vi "Puma Ground Control Station Read Version.vi"() -> ()   [LabVIEW 2014]
doc: "The Advanced Serial Read and Write example performs a Serial Port Read, a Serial Port Write, or a combination of these actions while setting some advanced serial features like buffer size, termination characters, and XON/XOFF flow control. The user selects the actions (read or write) on the front panel. If both are selected, the VI will write the data first, read the data and then close the VISA session that is opened to the port. \n\nThe parameters set for the serial port must match the parameters of the connected instrument or device. In this example, the bytes to read parameter specifies the number of bytes that the serial port reads. If there were more bytes at the port than the number specified in bytes to read, those bytes would not be read. Also, if you specify to read more bytes than the number of bytes actually read, you might receive a timeout error message.\n\nINSTRUCTIONS:\n1) Select the serial resource and configuration parameters (baud rate, data bits, parity, stop bits, flow control).\n2) Termination character can be enabled and set. Also, set the required input buffer size prior to running the example.\n3) Select the operations to be performed. \n4) Connect the serial port to your device. If no device is available, perform a loopback test by doing one of the following. Short pins 2 and 3 on a RS-232 cable or short pin 4 to pin 8 and pin 5 to pin 9 on a RS-485/422 cable. \n5) Run the VI to see the data read. (The \"read string\" will match the \"string to write\" if a loopback test was performed.)\n\nThis example exposes several advanced features that you may need for your application. Not all applications need all the features shown in this example. The input buffer size is likely an important setting that you want to control in your application. This example expands upon the flow control option for XON and XOFF, allowing the user to choose those control characters. The timeout parameter has been brought to the front panel so a user can specify the time period the VISA Read will wait for the number of bytes to read before timing out. Also, the user has several controls for the termination character, which is discussed later.\n\nNote that you can press the write and read buttons and change the bytes to read parameters on the fly, while the example is running. However, you must stop the example to change the other configuration parameters after the example has started running, and then run again.\n\nSet the I/O buffer size slightly higher the amount of data you expect to receive. This is very important for applications that don't use flow control, as you may lose characters if the receive buffer overflows.\n\nSetting the timeout period ensures that the operation returns with a timeout error if the operation cannot be performed in the specified time period. \n\nSome devices require a termination character in order to identify the end of command strings. Some devices send a termination character to signify the end of data to be read. \n\nThis example shows how you can end the Read operation once a termination character is detected in the buffer and/or append a termination character at the end of the Write data. To enable the Read to end on a termination character, use the VISA Configure Serial Port or use the VISA Properties Serial End Mode for Reads, Termination Character Enable, and Termination Character. To end the Write with a termination character, use the VISA Properties Serial End Mode for Writes, the Send End Enable, and Termination Character. In this example, the same termination character is used for both the Read and the Write. You can specify two different characters for your application, if desired.\n\nYour application may require specific characters for the XON/XOFF Flow Control. You can specify these characters with the VISA Properties Flow Control XOFF Character and Flow Control XON Character. Note that if the standard XON and XOFF characters are used, then decimal 17 and 19 are unavailable for data values. Remember that using flow control and setting an adequate buffer size allow you to prevent buffer overflows."
panel:
  out "soft kill ind":bool
  out "dump fuel ind":bool
  out "abort ind":bool
  out "run ind":bool
  out "av6-t ind":bool
  out "Control input":bool
  out "return yes on a completed input":bool
  out "Control (on/off)":bool
  out "PT 7":dbl
  out "PT7":dbl
  out "PT6":dbl
  out "PT5":dbl
  out "PT4":dbl
  out "PT3":dbl
  out "PT2":dbl
  out "PT1":dbl
  out "TC6":dbl
  out "TC5":dbl
  out "TC4":dbl
  out "TC3":dbl
  out "TC2":dbl
  out "TC1":dbl
  out "Output":string
  in  "?":enum32{"Check Out's", "Test"}(tab)
  in  "Tank ISO / AV5-T":bool
  in  "DValve / AV6-T":bool
  in  "Ullage ISO / FC-U":bool
  in  "Safety":bool
  in  "Test Run":bool
  in  "Reset Control":bool
  out "?":bool
  out "?":bool
  out "?":bool
  out "?":bool
  in  "Soft Kill":bool
  in  "Reset FC":bool
  in  "Safety":bool
  in  "Takeoff":bool
  in  "abort":bool
  out "?":dbl(graph)
  out "?":string[](array[string])
  out "?":string[](array[string])
  out "?":T1(graph)
  out "Voltage Sensor":dbl
  out "PT 1":dbl
  out "PT 2":dbl
  out "PT 3":dbl
  out "PT 4":dbl
  out "PT 5":dbl
  out "PT 6":dbl
  out "TC 1":dbl
  out "TC 2":dbl
  out "TC 3":dbl
  out "TC 4":dbl
  out "TC 5":dbl
  out "TC 6":dbl
  in  "dump fuel":bool
  in  "?":enum32{"PT", "TC", "Test"}(tab)
  in  "?":T2(tab)
  out "PT 1":dbl(graph)
  out "PT 2":dbl(graph)
  out "PT 3":dbl(graph)
  out "PT 4":dbl(graph)
  out "PT 5":dbl(graph)
  out "PT 6":dbl(graph)
  out "PT 7":dbl(graph)
  in  "?":T3(tab)
  out "TC 1":dbl(graph)
  out "TC 2":dbl(graph)
  out "TC 3":dbl(graph)
  out "TC 4":dbl(graph)
  out "TC 5":dbl(graph)
  out "TC 6":dbl(graph)
  out "?":bool
  out "String":string
  in  "String 3":string
  in  "Turn Off":bool
  in  "?":bool
  in  "Av-6Tt":bool
  in  "?":bool
  out "AV4-T":bool
  out "AV3-T":bool
  out "AV2-T":bool
  out "AV1-T":bool
  out "AV6-T":bool
  out "AV5-T":bool
  out "FO-U":bool
  out "FC-U":bool
  out "?":dbl(slide) scale=0.2..200.0
  # "FC-U"
  # "FO-U"
  # "AV1-T"
  # "AV2-T"
  # "AV3-T"
  # "AV4-T"
  # "AV5-T"
  # "AV6-T"
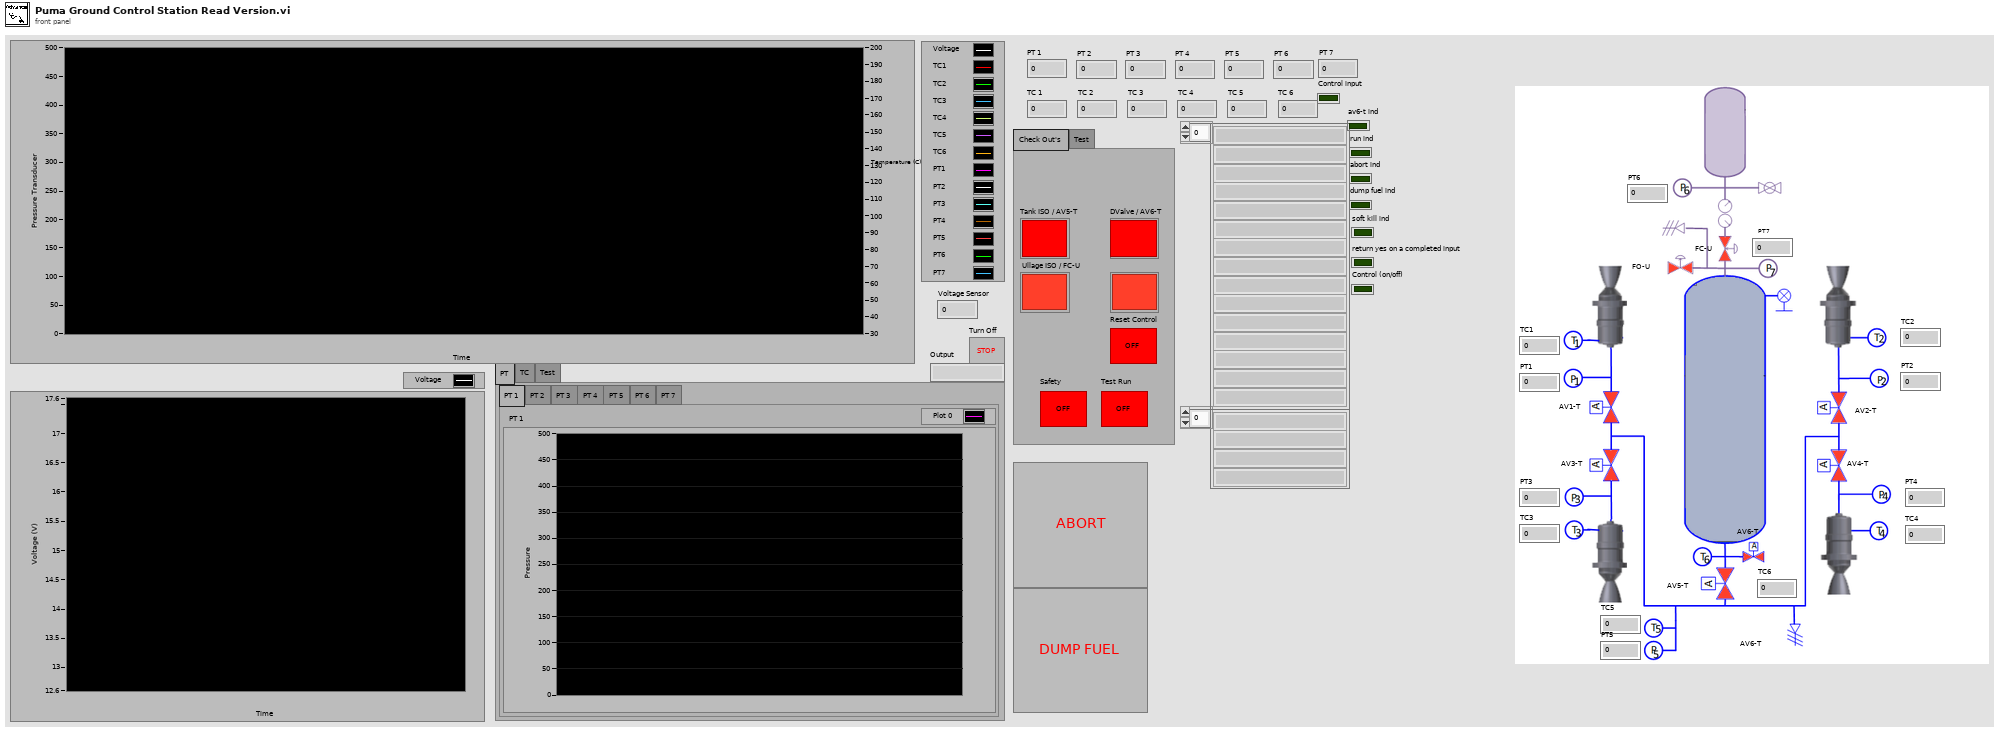
[diagram p1: front panel]
types:
  T1 = cluster{dbl, dbl, dbl, dbl, dbl, dbl, dbl, dbl, dbl, dbl, dbl, dbl, dbl, dbl}
  T2 = enum32{"PT 1", "PT 2", "PT 3", "PT 4", "PT 5", "PT 6", "PT 7"}
  T3 = enum32{"TC 1", "TC 2", "TC 3", "TC 4", "TC 5", "TC 6"}
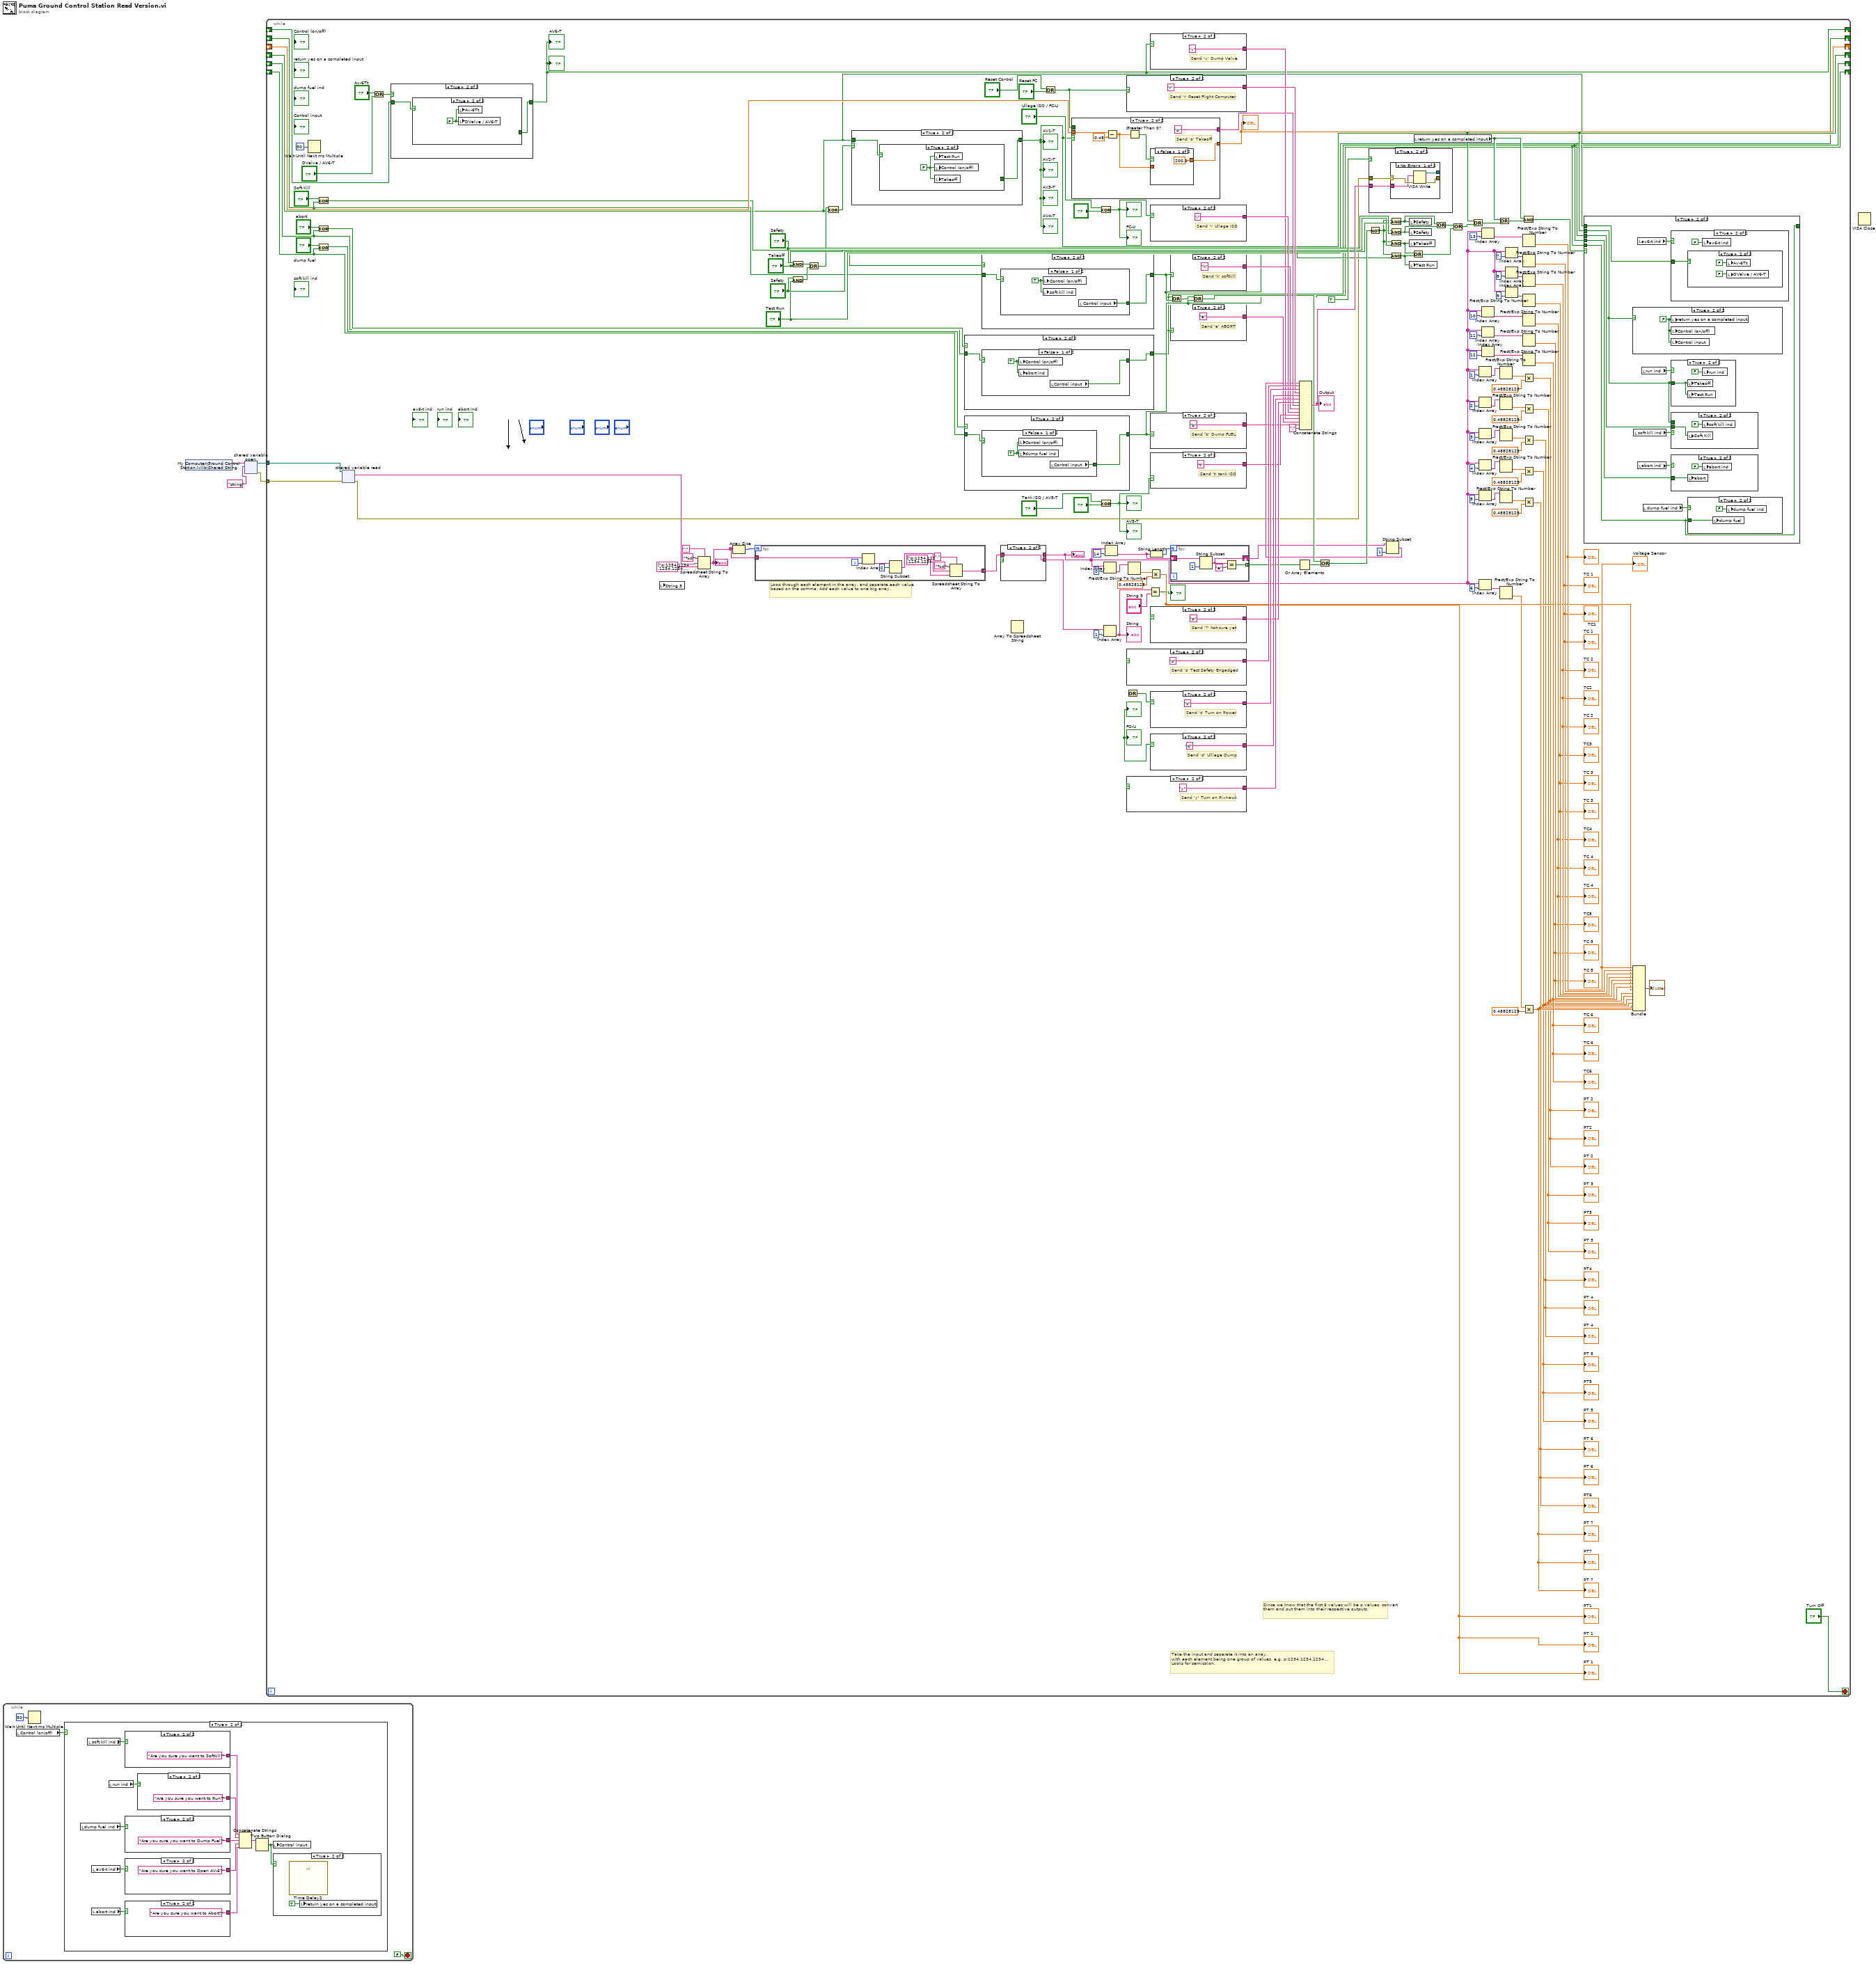
[diagram p0: block diagram]
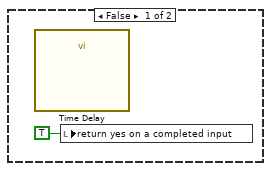
[diagram p8: hidden frame]
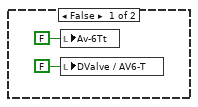
[diagram p11: hidden frame]
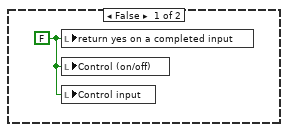
[diagram p16: hidden frame]
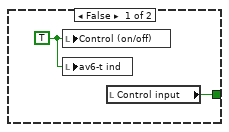
[diagram p18: hidden frame]
diagram:
  n1 = while {
    stop <- FALSE stop-if-true
    n2 = local read "Control (on/off)"() -> (w7:bool)
    n3 = Wait Until Next ms Multiple(millisecond multiple=u32 50 ("milliseconds to wait")) -> ()  [unwired: 1 out]
    n4 = case shown="True" w7 {
      frame False {
      }
      frame True {
        n5 = local read "dump fuel ind"() -> (w16:bool)
        n6 = local read "soft kill ind"() -> (w14:bool)
        n7 = local read "av6-t ind"() -> (w17:bool)
        n8 = local read "abort ind"() -> (w18:bool)
        n9 = local read "run ind"() -> (w15:bool)
        n10 = case shown="True" w14 {
          tunnel: [_ "Are you sure you want to Softkill?"] -> w9
          frame False {
          }
          frame True {
          }
        }
        n11 = case shown="True" w16 {
          tunnel: [_ "Are you sure you want to Dump Fuel?"] -> w11
          frame False {
          }
          frame True {
          }
        }
        n12 = case shown="True" w17 {
          tunnel: [_ "Are you sure you want to Open AV-6?"] -> w12
          frame False {
          }
          frame True {
          }
        }
        n13 = case shown="True" w18 {
          tunnel: [_ "Are you sure you want to Abort?"] -> w13
          frame False {
          }
          frame True {
          }
        }
        n14 = case shown="True" w15 {
          tunnel: [_ "Are you sure you want to Run?"] -> w10
          frame False {
          }
          frame True {
          }
        }
        n15 = Concatenate Strings(w9, w10, w11, w12, w13) -> (w8:string)
        n16 = Two Button Dialog(message=w8) -> (T button?=w19:bool)  [unwired: 2 in]
        n17 = local write "Control input"(w19) -> ()
        n18 = case shown="True" w19 {
          frame False {
            n19 = call "Time Delay"() -> ()  [unwired: 11 in, 1 out]
            n20 = local write "return yes on a completed input"(TRUE) -> ()
          }
          frame True {
            n21 = call "Time Delay2"() -> ()  [unwired: 11 in, 1 out]
            n22 = local write "return yes on a completed input"(TRUE) -> ()
          }
        }
      }
    }
  }
  n23 = shared-variable "My Computer\\Ground Control Station.lvlib\\Shared String"() -> (w4:string)  [unwired: 1 in, 1 out]
  n24 = shared-variable-open(w4, "string") -> (w2:refnum<k21>, w1:errorcluster)  [unwired: 2 in]
  n25 = while {
    shift-right: [w115] -> _
    shift-left: _ -> [w114]
    shift-right: [w56] -> _
    shift-left: _ -> [w38]
    shift-right: [w46] -> _
    shift-left: _ -> [w47]
    shift-right: [w36] -> _
    shift-left: _ -> [w63]
    shift-right: [w37] -> _
    shift-left: _ -> [w60]
    shift-right: [w39] -> _
    shift-left: _ -> [w42]
    tunnel: w2 -> [w30]
    tunnel: w1 -> [w27]
    stop <- "Turn Off" stop-if-true
    # "Since we know that the first 6 values will be p values, convert them and put them into their respective outputs."
    # "Loop through each element in the array, and separate each value\nbased on the comma. Add each value to one big array."
    # "Take the input and separate it into an array,\nwith each element being one group of values, e.g. p:1234,1234,1234...\nLooks for semicolon."
    n26 = Wait Until Next ms Multiple(millisecond multiple=u32 50 ("milliseconds to wait")) -> ()  [unwired: 1 out]
    n27 = Exclusive Or(1:w42, 2:"Soft Kill") -> (0:w40:bool)
    n28 = Exclusive Or(1:w63, 2:"abort") -> (0:w65:bool)
    n29 = Exclusive Or(1:w60, 2:"dump fuel") -> (0:w62:bool)
    n30 = shared-variable-read(w30, w27) -> (w28:errorcluster, w29:string)  [unwired: 2 out]
    n31 = Or(x="Av-6Tt", y="DValve / AV6-T") -> (x .or. y?=w43:bool)
    n32 = case shown="True" w43 {
      tunnel: [w207 w208] -> w46
      tunnel: w47 -> [w207 w209]
      frame False {
      }
      frame True {
        n33 = case shown="True" w209 {
          tunnel: [w211 _] -> w208
          frame False {
            w210 = TRUE
            n34 = local write "Control (on/off)"(w210) -> ()
            n35 = local write "av6-t ind"(w210) -> ()
            n36 = local read "Control input"() -> (w211:bool)
          }
          frame True {
            w212 = FALSE
            n37 = local write "Av-6Tt"(w212) -> ()
            n38 = local write "DValve / AV6-T"(w212) -> ()
          }
        }
      }
    }
    "AV6-T" <- w46
    "?" <- w46
    n39 = local read "String 3"() -> ()  [unwired: 1 in]
    n40 = Spreadsheet String To Array(delimiter (Tab)=";", format string="%d", spreadsheet string=w29, array type (2D Dbl)=string[] ["p:1234.1234.1234.1234,1234,1234", "t:1234,1234,1234"] ("Array of Strings 3")) -> (array=w173:string[])
    "?" <- w173
    n41 = Array Size(array=w173) -> (size(s)=w174:i32)
    n42 = for {
      N: w174 -> [_]
      tunnel: w173 -> [w282]
      tunnel: [w274] -> w84 mode=concatenating
      i -> [w281]
      n43 = Index Array(array=w282, index=w281) -> (element=w277:string)
      n44 = String Subset(string=w277, offset (0)=2) -> (substring=w275:string)  [unwired: 1 in]
      n45 = Spreadsheet String To Array(delimiter (Tab)=",", format string="%d", spreadsheet string=w275, array type (2D Dbl)=string[] ["p:1234.1234.1234.1234,1234,1234", "t:1234,1234,1234"] ("Array of Strings 3")) -> (array=w274:string[])
    }
    n46 = And(x="Safety", y="Takeoff") -> (x .and. y?=w133:bool)
    n47 = And(x="Safety", y="Test Run") -> (x .and. y?=w134:bool)
    n48 = Or(x=w133, y=w134) -> (x .or. y?=w68:bool)
    n49 = Exclusive Or(1:w38, 2:w68) -> (0:w67:bool)
    n50 = case shown="True" w67 {
      tunnel: [w229 w231] -> w56
      tunnel: w38 -> [w229 w230]
      frame False {
      }
      frame True {
        n51 = case shown="True" w230 {
          tunnel: [w233 _] -> w231
          frame False {
            w232 = TRUE
            n52 = local write "Control (on/off)"(w232) -> ()
            n53 = local write "run ind"(w232) -> ()
            n54 = local read "Control input"() -> (w233:bool)
          }
          frame True {
            w234 = FALSE
            n55 = local write "Test Run"(w234) -> ()
            n56 = local write "Control (on/off)"(w234) -> ()
            n57 = local write "Takeoff"(w234) -> ()
          }
        }
      }
    }
    "AV1-T" <- w56
    "AV4-T" <- w56
    "AV2-T" <- w56
    "AV3-T" <- w56
    n58 = case shown="True" w65 {
      tunnel: [w223 w225] -> w36
      tunnel: w63 -> [w223 w224]
      frame False {
      }
      frame True {
        n59 = case shown="False" w224 {
          tunnel: [w226 FALSE ("T button?")] -> w225
          frame False {
            w227 = TRUE
            n60 = local write "Control (on/off)"(w227) -> ()
            n61 = local write "abort ind"(w227) -> ()
            n62 = local read "Control input"() -> (w226:bool)
          }
          frame True {
          }
        }
      }
    }
    n63 = case shown="True" w62 {
      tunnel: [w218 w220] -> w37
      tunnel: w60 -> [w218 w219]
      frame False {
      }
      frame True {
        n64 = case shown="False" w219 {
          tunnel: [w222 _] -> w220
          frame False {
            w221 = TRUE
            n65 = local write "Control (on/off)"(w221) -> ()
            n66 = local write "dump fuel ind"(w221) -> ()
            n67 = local read "Control input"() -> (w222:bool)
          }
          frame True {
          }
        }
      }
    }
    n68 = case shown="True" w40 {
      tunnel: [w213 w215] -> w39
      tunnel: w42 -> [w213 w214]
      frame False {
      }
      frame True {
        n69 = case shown="False" w214 {
          tunnel: [w216 _] -> w215
          frame False {
            w217 = TRUE
            n70 = local write "Control (on/off)"(w217) -> ()
            n71 = local write "soft kill ind"(w217) -> ()
            n72 = local read "Control input"() -> (w216:bool)
          }
          frame True {
          }
        }
      }
    }
    n73 = case shown="True" {
      selector: _ -> [_ _]
      tunnel: w84 -> [w240 w241]
      tunnel: [w240 _] -> w85
      tunnel: [_ w241] -> w83
      frame False {
      }
      frame True {
      }
    }
    "?" <- w85
    n74 = Array To Spreadsheet String() -> ()  [unwired: 3 in, 1 out]
    n75 = Or(x="Reset Control", y="Reset FC") -> (x .or. y?=w116:bool)
    n76 = case shown="True" w56 {
      tunnel: [_ "o" ("write buffer")] -> w138
      tunnel: w114 -> [w251 w259]
      tunnel: [w252 w255] -> w115
      tunnel: w116 -> [w250 _]
      frame False {
        n77 = case shown="False" w250 {
          tunnel: [w253 200.0] -> w252
          tunnel: w251 -> [w253 _]
          frame False {
          }
          frame True {
          }
        }
      }
      frame True {
        # "Send 'o' Takeoff"
        n78 = Subtract(x=w259, y=0.48) -> (x-y=w256:dbl)
        n79 = Greater Than 0?(x=w256) -> (x > 0?=w257:bool)
        n80 = case shown="False" w257 {
          tunnel: w256 -> [_ w262]
          tunnel: [200.0 w262] -> w255
          frame False {
          }
          frame True {
          }
        }
      }
    }
    "?" <- w115
    n81 = Exclusive Or(1:"?", 2:"Ullage ISO / FC-U") -> (0:w107:bool)
    "FC-U" <- w107
    "?" <- w107
    n82 = Exclusive Or(1:"?", 2:"Tank ISO / AV5-T") -> (0:w110:bool)
    "AV5-T" <- w110
    "?" <- w110
    n83 = Index Array(array=w85, index=0) -> (element=w166:string)
    n84 = Index Array(array=w83, index=1) -> (element=w82:string)
    "String" <- w82
    n85 = Index Array(array=w85, index=14) -> (element=w31:string)
    n86 = case shown="True" w116 {
      tunnel: [_ "r" ("write buffer")] -> w142
      frame False {
      }
      frame True {
        # "Send 'r' Reset Flight Computer"
      }
    }
    n87 = case shown="True" {
      selector: _ -> [_ _]
      tunnel: [_ "s" ("write buffer")] -> w145
      frame False {
      }
      frame True {
        # "Send 's' Test Safety Engadged"
      }
    }
    n88 = case shown="True" {
      selector: _ -> [_ _]
      tunnel: [_ "y" ("write buffer")] -> w140
      frame False {
      }
      frame True {
        # "Send 'y' Turn on Pixhawk"
      }
    }
    n89 = Or() -> (x .or. y?=w132:bool)  [unwired: 2 in]
    n90 = Fract/Exp String To Number(string=w166) -> (number=w102:dbl)  [unwired: 3 in, 1 out]
    n91 = Equal?(x=w82, y="String 3") -> (x = y?=→"?":bool)
    n92 = Multiply(x=w102, y=0.48828125) -> (x*y=w101:dbl)
    "PT 1" <- w101
    "PT 1" <- w101
    "PT1" <- w101
    n93 = case shown="True" w46 {
      tunnel: [_ "v" ("write buffer")] -> w128
      frame False {
      }
      frame True {
        # "Send 'v' Dump Valve"
      }
    }
    n94 = case shown="True" w107 {
      tunnel: [_ "i" ("write buffer")] -> w130
      frame False {
      }
      frame True {
        # "Send 'i' Ullage ISO"
      }
    }
    n95 = case shown="True" w37 {
      tunnel: [_ "b" ("write buffer")] -> w127
      frame False {
      }
      frame True {
        # "Send 'b' Dump FUEL"
      }
    }
    n96 = case shown="True" w110 {
      tunnel: [_ "t" ("write buffer")] -> w129
      frame False {
      }
      frame True {
        # "Send 't' tank ISO"
      }
    }
    n97 = String Length(string=w31) -> (length=w78:i32)
    n98 = case shown="True" {
      selector: _ -> [_ _]
      tunnel: [_ "p" ("write buffer")] -> w139
      frame False {
      }
      frame True {
        # "Send '?' Not sure yet"
      }
    }
    n99 = case shown="True" w132 {
      tunnel: [_ "z" ("write buffer")] -> w143
      frame False {
      }
      frame True {
        # "Send 'z' Turn on Power"
      }
    }
    n100 = case shown="True" "?" {
      tunnel: [_ "d" ("write buffer")] -> w131
      frame False {
      }
      frame True {
        # "Send 'd' Ulliage Dump"
      }
    }
    n101 = case shown="True" w39 {
      tunnel: [_ "k" ("write buffer")] -> w141
      frame False {
      }
      frame True {
        # "Send 'k' softkill"
      }
    }
    n102 = Or(x=w36, y=w39) -> (x .or. y?=w66:bool)
    n103 = case shown="True" w36 {
      tunnel: [_ "a" ("write buffer")] -> w126
      frame False {
      }
      frame True {
        # "Send 'a' ABORT"
      }
    }
    n104 = for {
      N: w78 -> [_]
      shift-right: [w237] -> w33
      shift-left: w31 -> [w236]
      tunnel: [w235] -> w77 mode=indexing
      n105 = String Subset(string=w236, length (rest)=1 ("length (rest)")) -> (substring=w237:string)  [unwired: 1 in]
      n106 = Equal?(x=w237, y="e") -> (x = y?=w235:bool)
    }
    n107 = Or(x=w66, y=w37) -> (x .or. y?=w75:bool)
    n108 = Or Array Elements(Boolean array=w77) -> (logical OR=w76:bool)
    n109 = Or(x=w75, y=w76) -> (x .or. y?=w74:bool)
    n110 = Not(x=w74) -> (.not. x?=w70:bool)
    n111 = String Subset(string=w33, length (rest)=1 ("length (rest)")) -> (substring=w35:string)  [unwired: 1 in]
    n112 = Concatenate Strings(w35, w145, w143, w142, w131, w140, w139, w138, w141, w130, w129, w128, w126, w127, ";" ("string")) -> (w137:string)
    "Output" <- w137
    n113 = case shown="True" TRUE {
      tunnel: w137 -> [_ w268]
      tunnel: w28 -> [_ w267]
      frame False {
      }
      frame True {
        n114 = case shown="No Error" w267 {
          selector: w267 -> [w270 w273]
          tunnel: [w272 _] -> _
          tunnel: [w271 w273] -> _
          tunnel: w268 -> [w269 _]
          frame No Error {
            n115 = VISA Write(write buffer=w269, error in (no error)=w270) -> (VISA resource name out=w272:refnum<visa-resource-name>, error out=w271:errorcluster)  [unwired: 1 in, 1 out]
          }
          frame Error {
          }
        }
      }
    }
    n116 = And(x=w70, y="Safety") -> (x .and. y?=w51:bool)
    n117 = And(x=w70, y="Safety") -> (x .and. y?=w50:bool)
    n118 = And(x=w70, y="Takeoff") -> (x .and. y?=w49:bool)
    n119 = And(x=w70, y="Test Run") -> (x .and. y?=w48:bool)
    n120 = local write "Safety"(w51) -> ()
    n121 = local write "Safety"(w50) -> ()
    n122 = local write "Takeoff"(w49) -> ()
    n123 = local write "Test Run"(w48) -> ()
    n124 = Or(x=w49, y=w48) -> (x .or. y?=w53:bool)
    n125 = local read "return yes on a completed input"() -> (w58:bool)
    n126 = Or(x=w51, y=w50) -> (x .or. y?=w54:bool)
    n127 = Or(x=w54, y=w53) -> (x .or. y?=w52:bool)
    n128 = Or(x=w56, y=w52) -> (x .or. y?=w55:bool)
    n129 = Index Array(array=w85, index=1) -> (element=w165:string)
    n130 = Index Array(array=w85, index=2) -> (element=w164:string)
    n131 = Index Array(array=w85, index=3) -> (element=w163:string)
    n132 = Index Array(array=w85, index=4) -> (element=w162:string)
    n133 = Index Array(array=w85, index=5) -> (element=w161:string)
    n134 = Index Array(array=w85, index=6) -> (element=w118:string)
    n135 = Index Array(array=w85, index=13) -> (element=w147:string)
    n136 = Index Array(array=w85, index=10) -> (element=w151:string)
    n137 = Index Array(array=w85, index=11) -> (element=w150:string)
    n138 = Index Array(array=w85, index=12) -> (element=w149:string)
    n139 = Or(x=w58, y=w55) -> (x .or. y?=w59:bool)
    n140 = Fract/Exp String To Number(string=w165) -> (number=w87:dbl)  [unwired: 3 in, 1 out]
    n141 = Fract/Exp String To Number(string=w164) -> (number=w90:dbl)  [unwired: 3 in, 1 out]
    n142 = Fract/Exp String To Number(string=w163) -> (number=w93:dbl)  [unwired: 3 in, 1 out]
    n143 = Fract/Exp String To Number(string=w162) -> (number=w96:dbl)  [unwired: 3 in, 1 out]
    n144 = Fract/Exp String To Number(string=w161) -> (number=w105:dbl)  [unwired: 3 in, 1 out]
    n145 = Fract/Exp String To Number(string=w118) -> (number=w99:dbl)  [unwired: 3 in, 1 out]
    n146 = Index Array(array=w85, index=7) -> (element=w155:string)
    n147 = Index Array(array=w85, index=8) -> (element=w154:string)
    n148 = Index Array(array=w85, index=9) -> (element=w153:string)
    n149 = And(x=w58, y=w59) -> (x .and. y?=w57:bool)
    n150 = Fract/Exp String To Number(string=w147) -> (number=w146:dbl)  [unwired: 3 in, 1 out]
    "Voltage Sensor" <- w146
    "?" <- w146
    n151 = Fract/Exp String To Number(string=w155) -> (number=w119:dbl)  [unwired: 3 in, 1 out]
    "TC 1" <- w119
    "TC 1" <- w119
    "TC1" <- w119
    n152 = Fract/Exp String To Number(string=w154) -> (number=w124:dbl)  [unwired: 3 in, 1 out]
    "TC 2" <- w124
    "TC 2" <- w124
    "TC2" <- w124
    n153 = Fract/Exp String To Number(string=w153) -> (number=w123:dbl)  [unwired: 3 in, 1 out]
    "TC 3" <- w123
    "TC 3" <- w123
    "TC3" <- w123
    n154 = Fract/Exp String To Number(string=w151) -> (number=w122:dbl)  [unwired: 3 in, 1 out]
    "TC 4" <- w122
    "TC 4" <- w122
    "TC4" <- w122
    n155 = Fract/Exp String To Number(string=w150) -> (number=w121:dbl)  [unwired: 3 in, 1 out]
    "TC 5" <- w121
    "TC 5" <- w121
    "TC5" <- w121
    n156 = Fract/Exp String To Number(string=w149) -> (number=w120:dbl)  [unwired: 3 in, 1 out]
    "TC 6" <- w120
    "TC 6" <- w120
    "TC6" <- w120
    n157 = Multiply(x=w87, y=0.48828125) -> (x*y=w86:dbl)
    "PT 2" <- w86
    "PT 2" <- w86
    "PT2" <- w86
    n158 = Multiply(x=w90, y=0.48828125) -> (x*y=w89:dbl)
    "PT 3" <- w89
    "PT 3" <- w89
    "PT3" <- w89
    n159 = Multiply(x=w93, y=0.48828125) -> (x*y=w92:dbl)
    "PT 4" <- w92
    "PT 4" <- w92
    "PT4" <- w92
    n160 = Multiply(x=w96, y=0.48828125) -> (x*y=w95:dbl)
    "PT 5" <- w95
    "PT 5" <- w95
    "PT5" <- w95
    n161 = Multiply(x=w105, y=0.48828125) -> (x*y=w104:dbl)
    "PT 6" <- w104
    "PT 6" <- w104
    "PT6" <- w104
    n162 = Multiply(x=w99, y=0.48828125) -> (x*y=w98:dbl)
    "PT7" <- w98
    "PT 7" <- w98
    "PT 7" <- w98
    n163 = case shown="True" w57 {
      tunnel: w56 -> [_ w182]
      tunnel: w39 -> [_ w185]
      tunnel: w38 -> [_ w184]
      tunnel: [_ w183] -> _
      tunnel: w37 -> [_ w183]
      tunnel: w36 -> [_ w181]
      frame False {
      }
      frame True {
        n164 = case shown="True" w182 {
          frame False {
            w205 = FALSE
            n165 = local write "return yes on a completed input"(w205) -> ()
            n166 = local write "Control (on/off)"(w205) -> ()
            n167 = local write "Control input"(w205) -> ()
          }
          frame True {
            w206 = FALSE
            n168 = local write "return yes on a completed input"(w206) -> ()
            n169 = local write "Control (on/off)"(w206) -> ()
            n170 = local write "Control input"(w206) -> ()
          }
        }
        n171 = local read "soft kill ind"() -> (w190:bool)
        n172 = local read "av6-t ind"() -> (w186:bool)
        n173 = local read "abort ind"() -> (w187:bool)
        n174 = local read "run ind"() -> (w188:bool)
        n175 = local read "dump fuel ind"() -> (w189:bool)
        n176 = case shown="True" w186 {
          tunnel: w184 -> [_ w192]
          frame False {
          }
          frame True {
            n177 = case shown="True" w192 {
              frame False {
                n178 = local write "Av-6Tt"(FALSE) -> ()
                n179 = local write "DValve / AV6-T"(FALSE) -> ()
              }
              frame True {
                n180 = local write "Av-6Tt"(FALSE) -> ()
                n181 = local write "DValve / AV6-T"(FALSE) -> ()
              }
            }
            n182 = local write "av6-t ind"(FALSE) -> ()
          }
        }
        n183 = case shown="True" w188 {
          tunnel: w182 -> [_ w204]
          frame False {
          }
          frame True {
            n184 = local write "Takeoff"(w204) -> ()
            n185 = local write "Test Run"(w204) -> ()
            n186 = local write "run ind"(FALSE) -> ()
          }
        }
        n187 = case shown="True" w190 {
          tunnel: w182 -> [_ _]
          tunnel: w185 -> [_ w199]
          frame False {
          }
          frame True {
            n188 = local write "Soft Kill"(w199) -> ()
            n189 = local write "soft kill ind"(FALSE) -> ()
          }
        }
        n190 = case shown="True" w187 {
          tunnel: w181 -> [_ w197]
          frame False {
          }
          frame True {
            n191 = local write "abort"(w197) -> ()
            n192 = local write "abort ind"(FALSE) -> ()
          }
        }
        n193 = case shown="True" w189 {
          tunnel: w183 -> [_ w201]
          frame False {
          }
          frame True {
            n194 = local write "dump fuel"(w201) -> ()
            n195 = local write "dump fuel ind"(FALSE) -> ()
          }
        }
      }
    }
    n196 = Bundle(w146, w119, w124, w123, w122, w121, w120, w101, w86, w89, w92, w95, w104, w98) -> (→"?":T1)  [unwired: 1 out]
    "FO-U" <- "?"
  }
  n197 = VISA Close() -> ()  [unwired: 2 in, 1 out]
